vi "Do.vi"(8 "error in (no error)":errorcluster, 10 "Actor in":refnum<class "Actor.lvclass">, 11 "New Results Msg":refnum<class "New Results Msg.lvclass">) -> (0 "error out":errorcluster, 2 "Actor out":refnum<class "Actor.lvclass">)   [LabVIEW 2014, in "POLARIS Target Focus Actor.lvlib" / "New Results Msg.lvclass"]
doc: "This VI delivers the message to the actor by calling the appropriate method(s) on the actor."
uses:
  New Results Msg.lvclass
  <vilib>/ActorFramework/Actor/Actor.lvclass
  POLARIS Target Focus Actor/POLARIS Target Focus Actor.lvclass
  Abstract Messages/Publish Analyze Results Msg/Publish Analyze Results Msg.lvclass/Publish Analyze Results Msg.ctl
  Abstract Messages/Publish Analyze Results Msg/Publish Analyze Results Msg.lvclass
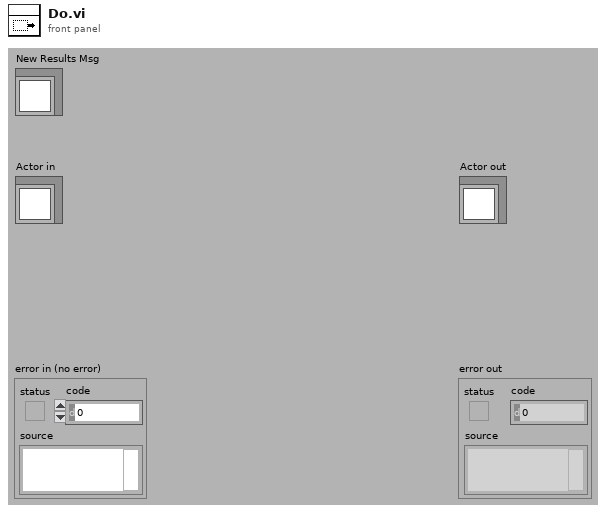
[diagram p1: front panel]
types:
  T1 = cluster{"Image Nr.":i32, "Results":refnum<class "Analyze Results Base.lvclass">[], "Parameters":refnum<class "Analyze Parameter Base.lvclass">[]}
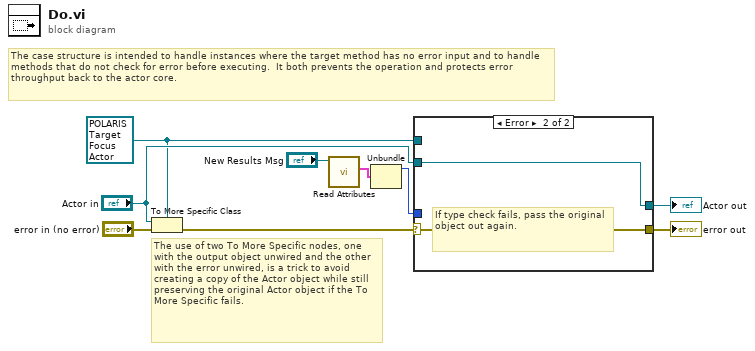
[diagram p0: block diagram]
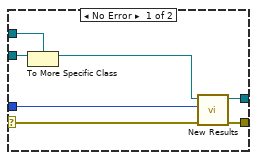
[diagram p2: hidden frame]
diagram:
  w4 = refnum<class "POLARIS Target Focus Actor.lvclass"> refnum ("Actor in")
  # "The use of two To More Specific nodes, one with the output object unwired and the other with the error unwired, is a trick to avoid creating a copy of the Actor object while still preserving the original Actor object if the To More Specific fails."
  # "The case structure is intended to handle instances where the target method has no error input and to handle methods that do not check for error before executing.  It both prevents the operation and protects error throughput back to the actor core."
  n1 = To More Specific Class(target class=w4, reference="Actor in", error in="error in (no error)") -> (error out=w8:errorcluster)  [unwired: 1 out]
  n2 = call "Read Attributes.vi"("Abstract Message Template in"="New Results Msg") -> ("Payload"=w2:T1)  [unwired: 9 in, 1 out]
  n3 = Unbundle(w2) -> ("Image Nr."=w1:i32)  [unwired: 2 out]
  n4 = case shown="Error" w8 {
    selector: w8 -> [w14 w18]
    tunnel: [w16 w18] -> w7
    tunnel: [w15 w17] -> w6
    tunnel: "Actor in" -> [w13 w17]
    tunnel: w4 -> [w12 _]
    tunnel: w1 -> [w11 _]
    frame No Error {
      n5 = To More Specific Class(target class=w12, reference=w13) -> (specific class reference=w10:refnum<class "POLARIS Target Focus Actor.lvclass">)  [unwired: 1 in, 1 out]
      n6 = call "New Results.vi"("error in (no error)"=w14, "Results"=w11, "POLARIS Target Focus Actor in"=w10) -> ("error out"=w16:errorcluster, "POLARIS Target Focus Actor out"=w15:refnum<class "POLARIS Target Focus Actor.lvclass">)  [unwired: 7 in]
    }
    frame Error {
      # "If type check fails, pass the original object out again."
    }
  }
  "error out" <- w7
  "Actor out" <- w6
